vi "in place graph operation.vi"() -> ()   [LabVIEW 2016]
panel:
  in  "row":i32
  in  "col":i32
  out "Intensity Graph":dbl[][](graph)
  in  "dont just est":bool
  in  "generate/modify":bool
  out "MB array est":dbl
  in  "inner size":i32
  in  "outer size":i32
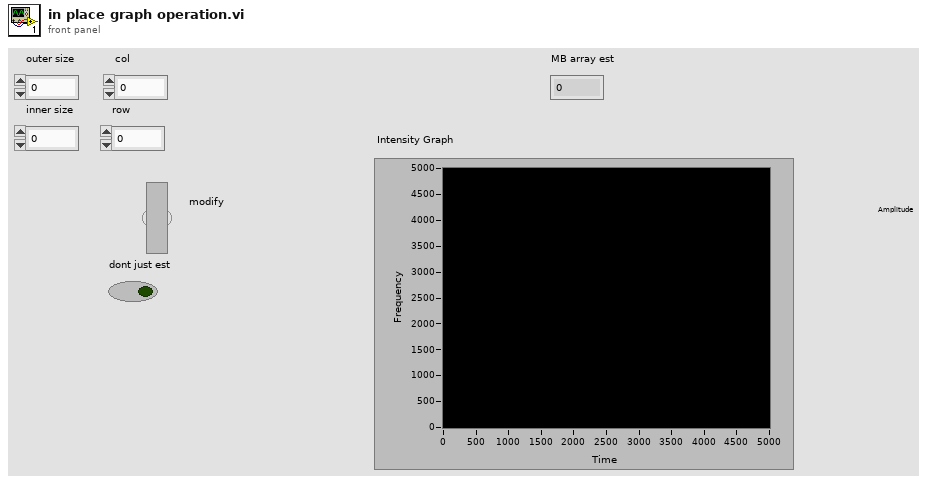
[diagram p1: front panel]
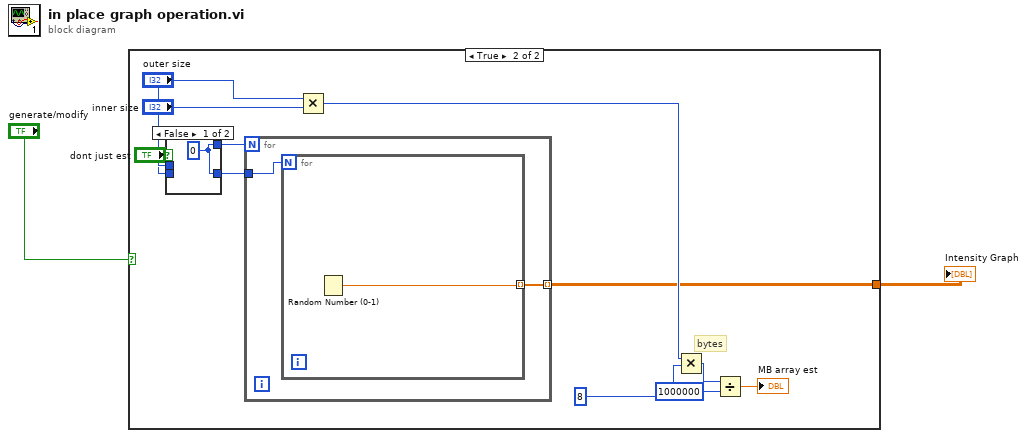
[diagram p0: block diagram]
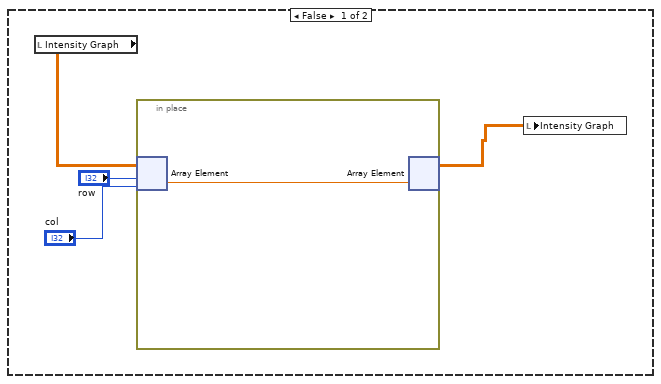
[diagram p2: hidden frame]
diagram:
  n1 = case shown="True" "generate/modify" {
    tunnel: [_ w8] -> w1
    frame False {
      n2 = local read "Intensity Graph"() -> (w3:dbl[][])
      n3 = in-place {
        n4 = in-place-array #1(w3, "row", "col") -> (w7:dbl)
        n5 = in-place-array #1(w7) -> (w4:dbl[][])  [unwired: 2 out]
      }
      n6 = local write "Intensity Graph"(w4) -> ()
    }
    frame True {
      # "bytes"
      n7 = case shown="False" "dont just est" {
        tunnel: "inner size" -> [_ w20]
        tunnel: "outer size" -> [_ w21]
        tunnel: [w19 w21] -> w11
        tunnel: [w19 w20] -> w10
        frame False {
          w19 = 0
        }
        frame True {
        }
      }
      n8 = for {
        N: w11 -> [_]
        tunnel: [w23] -> w8 mode=indexing
        tunnel: w10 -> [w22]
        n9 = for {
          N: w22 -> [_]
          tunnel: [w24] -> w23 mode=indexing
          n10 = Random Number (0-1)() -> (number: 0 to 1=w24:dbl)
        }
      }
      n11 = Multiply(x="outer size", y="inner size") -> (x*y=w14:i32)
      n12 = Multiply(x=w14, y=8) -> (x*y=w17:i32)
      n13 = Divide(x=w17, y=1000000) -> (x/y=→"MB array est":dbl)
    }
  }
  "Intensity Graph" <- w1
